vi "SV TDMS Read Spectrum (Waterfall).vi"(0 "tdms file":refnum<k34>, 5 "group name in":string="Spectrum_Waterfall", 11 "error in":errorcluster) -> (3 "scale labels":T1, 4 "tdms file out":refnum<k34>, 6 "group name out":string, 8 "channel names out":string[](array[string]), 10 "waterfall graph data":T2, 13 "spectrum info":T3 {"x-axis units" items=["Time (s)"=0, "Frequency-CB (Hz)"=1, "Frequency-CPB (Hz)"=1248, "Frequency-Arbitrary (Hz)"=2357, "Quefrency (s)"=2, "Revolutions (rev)"=3, "Order"=4, "Speed (RPM)"=11, "Speed (rad/s)"=21, "Index"=65535]; "weighting filter" items=["Linear", "A-weighting", "B-weighting", "C-weighting", "ITU-R 468-4", "Dolby", "CCITT", "C-message", "Wb", "Wc", "Wd", "We", "Wf", "Wh", "Wj", "Wk", "Wm", "AES17 20 kHz lowpass", "AES17 40 kHz lowpass", "AES17 20 kHz highpass", "AES17 40 kHz highpass"]; "dB reference [EU]" format="%.2f"; "engineering units" items=["custom..."=0, "V"=1, "A"=21, "C"=30, "pC"=31, "s"=32, "-"=29, "Pa"=2, "N"=20, "g"=3, "m/s^2"=4, "m/s"=5, "m"=6, "mm/s"=12, "mm"=13, "micron/s"=14, "micron"=15, "in/s^2"=7, "in/s"=8, "in"=9, "mil/s"=10, "mil"=11, "rad/s^2"=16, "rad/s"=17, "rad"=18, "deg/s^2"=26, "deg/s"=27, "deg"=28, "RPM"=22, "cycle/s^2"=23, "Hz"=24, "cycle"=25, "strain"=19]; "spectral info"."window" items=["None "=0, "Hanning"=1, "Hamming"=2, "Blackman-Harris"=3, "Exact Blackman"=4, "Blackman"=5, "Flat Top"=6, "4 Term B-Harris "=7, "7 Term B-Harris"=8, "Low Sidelobe"=9, "Force - Exponential"=10, "Gaussian"=62]}, 15 "error out":errorcluster)   [LabVIEW 2017]
doc: "Reads the specified .tdms file and returns data in a format specific to the polymorphic instance selected."
uses:
  <vilib>/addons/_NISVFA/_Shared subVIs/Controls/svc_Spectrum Info.ctl
  <vilib>/addons/_NISVFA/_Shared subVIs/Controls/svc_X-Axis Units.ctl
  <vilib>/addons/_NISVFA/_Shared subVIs/Controls/svc_Spectrum Type.ctl
  <vilib>/addons/_NISVFA/_Shared subVIs/Controls/svc_Engineering Units Text Ring.ctl
  <vilib>/addons/_NISVFA/_Shared subVIs/Controls/svc_Weighting Filter Text Ring.ctl
  <vilib>/addons/_NISVFA/_Shared subVIs/Controls/svc_Complimentary Spectrum Units.ctl
  <vilib>/addons/_NISVFA/_Shared subVIs/Controls/NI Channel Properties.ctl
  <vilib>/addons/_NISVFA/_Shared subVIs/Controls/LV Datatypes.ctl
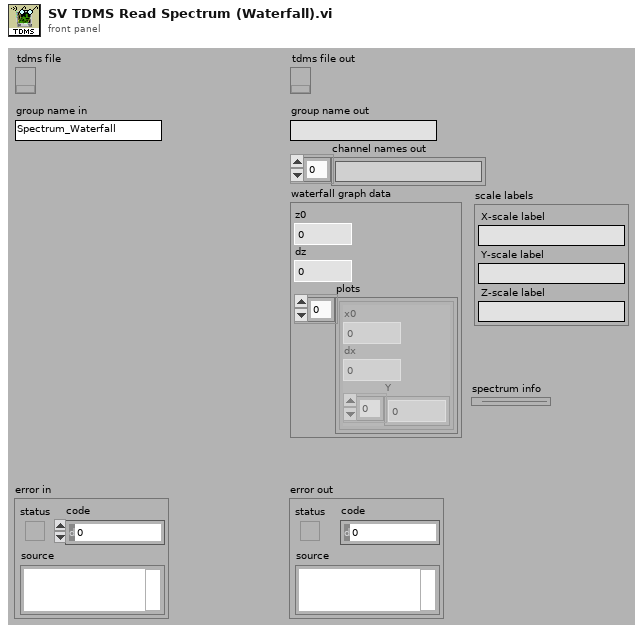
[diagram p1: front panel]
types:
  T1 = cluster{"X-scale label":string, "Y-scale label":string, "Z-scale label":string}
  T2 = cluster{"z0":dbl, "dz":dbl, "plots":cluster{"x0":dbl, "dx":dbl, "Y":dbl[]}[]}
  T3 = typedef "svc_Spectrum Info.ctl" = cluster{"channel name":string, "description":string, "x-axis units":T4, "spectral info":cluster{"spectrum type":T5, "linear/dB":enum16{"linear", "dB"}, "window":u16, "window size":i32, "FFT size":i32}, "engineering units":T6, "custom label":string, "dB reference [EU]":dbl, "peak units":enum16{"rms", "peak", "peak-peak"}, "weighting filter":T7, "spectral density?":bool, "unit label":string, "spectrum skewed?":bool, "complimentary spectrum units":T8}
  T4 = typedef "svc_X-Axis Units.ctl" = u16
  T5 = typedef "svc_Spectrum Type.ctl" = enum16{"FFT Spectrum [complex]", "Amplitude [Magnitude]", "Power [Magnitude^2]", "Cross Spectrum [complex]", "Frequency Response [Complex]"}
  T6 = typedef "svc_Engineering Units Text Ring.ctl" = u16
  T7 = typedef "svc_Weighting Filter Text Ring.ctl" = u16
  T8 = typedef "svc_Complimentary Spectrum Units.ctl" = enum16{"none", "radians", "degrees", "cycles", "imaginary"}
  T9 = typedef "LV Datatypes.ctl" = i32
  T10 = typedef "NI Channel Properties.ctl" = u16
  T11 = cluster{"X-scale label":string, "Y-scale label":string}
  T12 = cluster{"property values":dbl, "property values":dbl, cluster{"x0":dbl, "dx":dbl, "array":dbl[]}[]}
  T13 = cluster{"X-scale label":string, "Y-scale label":string, "scale label with units":string}
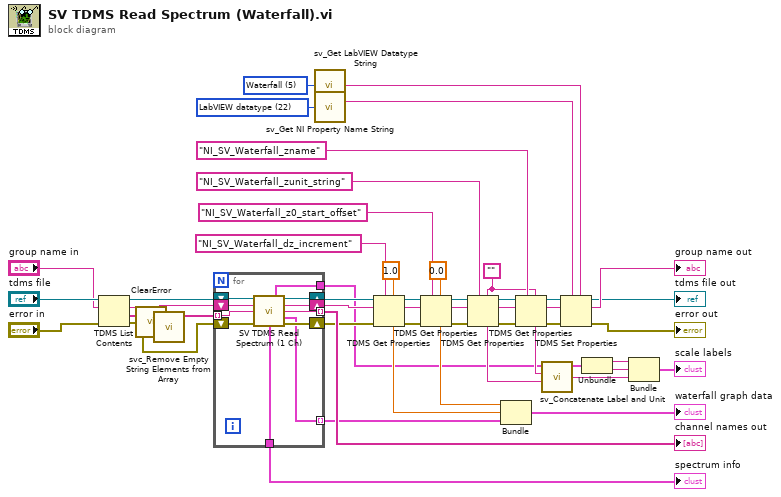
[diagram p0: block diagram]
diagram:
  w18 = "" ("channel name")
  w38 = T9 5 items=["String: abc"=-2, "Boolean: True or False"=-1, "Scalar: y"=0, "Array: Y"=1, "Waveform: t0, dt, Y, variant"=2, "Cluster: x0, dx, Y"=3, "Cluster: X, Y"=4, "Waterfall"=5, "Colormap"=6] ("LabVIEW datatype")
  w37 = T10 22 items=["Channel name", "Channel description", "Y-axis label", "Y-axis unit string", "X-axis label", "X-axis unit string", "x0", "dx", "Number of samples", "X channel", "Filter settled", "dB reference", "Window", "Window parameter", "Window size", "FFT size", "Peak units", "Spectrum type", "Magnitude scale", "Spectral density", "Sensor sensitivity (mV/EU)", "X-axis domain", "LabVIEW datatype"] ("property")
  n1 = TDMS List Contents(4:"error in", 6:"group name in", 7:"tdms file") -> (0:w1:errorcluster, 1:w2:string[], 2:w10:string, 3:w21:refnum<k34>)
  n2 = call <vilib>:"ClearError.vi"("error in (no error)"=w1) -> ("error out"=w3:errorcluster)
  n3 = call <vilib>:"svc_Remove Empty String Elements from Array.vi"("sparse array of strings"=w2) -> ("dense array of strings"=w4:string[])  [unwired: 10 in]
  n4 = for {
    shift-right: [w59] -> w27
    shift-left: w21 -> [w62]
    shift-right: [w57] -> w24
    shift-left: w3 -> [w61]
    shift-right: [w58] -> w23
    shift-left: w10 -> [w60]
    tunnel: [w56] -> w26
    tunnel: [w55] -> w25 mode=indexing
    tunnel: w4 -> [w54] mode=indexing
    tunnel: [w53] -> w14 mode=indexing
    tunnel: [w52] -> w7
    n5 = call <vilib>:"SV TDMS Read Spectrum (1 Ch).vi"("tdms file"=w62, "group name in"=w60, "channel name in"=w54, "error in"=w61) -> ("scale labels"=w52:T11, "tdms file out"=w59:refnum<k34>, "group name out"=w58:string, "channel name out"=w55:string, "spectrum"=w53:cluster{"x0":dbl, "dx":dbl, "array":dbl[]}, "spectrum info"=w56:T3, "error out"=w57:errorcluster)  [unwired: 5 in]
  }
  "channel names out" <- w25
  "spectrum info" <- w26
  n6 = call <vilib>:"sv_Get LabVIEW Datatype String.vi"("LabVIEW datatype"=w38) -> ("datatype string"=w30:string)  [unwired: 4 in]
  n7 = call <vilib>:"sv_Get NI Property Name String.vi"("property"=w37) -> ("TDMS property name"=w31:string)  [unwired: 13 in, 1 out]
  n8 = TDMS Get Properties(5:1.0 ("property values"), 7:"NI_SV_Waterfall_dz_increment" ("channel name"), 8:w24, 10:w23, 11:w27) -> (0:w43:errorcluster, 2:w44:string, 3:w45:refnum<k34>, 4:w15:dbl)  [unwired: 1 in, 2 out]
  n9 = TDMS Get Properties(5:0.0 ("property values"), 7:"NI_SV_Waterfall_z0_start_offset" ("channel name"), 8:w43, 10:w44, 11:w45) -> (0:w48:errorcluster, 2:w49:string, 3:w50:refnum<k34>, 4:w16:dbl)  [unwired: 1 in, 2 out]
  n10 = TDMS Get Properties(5:w18, 7:"NI_SV_Waterfall_zunit_string" ("channel name"), 8:w48, 10:w49, 11:w50) -> (0:w42:errorcluster, 2:w41:string, 3:w40:refnum<k34>, 4:w11:string)  [unwired: 1 in, 2 out]
  n11 = Bundle("property values"=w16, "property values"=w15, w14) -> (→"waterfall graph data":T12)  [unwired: 1 in]
  n12 = TDMS Get Properties(5:w18, 7:"NI_SV_Waterfall_zname" ("channel name"), 8:w42, 10:w41, 11:w40) -> (0:w36:errorcluster, 2:w35:string, 3:w34:refnum<k34>, 4:w12:string)  [unwired: 1 in, 2 out]
  n13 = call <vilib>:"sv_Concatenate Label and Unit.vi"("unit string"=w11, "label"=w12) -> ("scale label with units"=w9:string)  [unwired: 4 in]
  n14 = TDMS Set Properties(5:w30, 7:w31, 8:w36, 10:w35, 11:w34) -> (0:→"error out":errorcluster, 2:→"group name out":string, 3:→"tdms file out":refnum<k34>)  [unwired: 1 in, 1 out]
  n15 = Unbundle(w7) -> ("X-scale label"=w8:string, "Y-scale label"=w6:string)
  n16 = Bundle("X-scale label"=w8, "Y-scale label"=w6, "scale label with units"=w9) -> (→"scale labels":T13)  [unwired: 1 in]
